vi "Data Queue Single.vi"(7 "Action":T1(ring), 8 "error in (no error)":errorcluster, 11 "Data In":sgl[][](array[numeric])) -> (0 "error out":errorcluster, 3 "Data Out":sgl[][](array[numeric]))   [LabVIEW 2017]
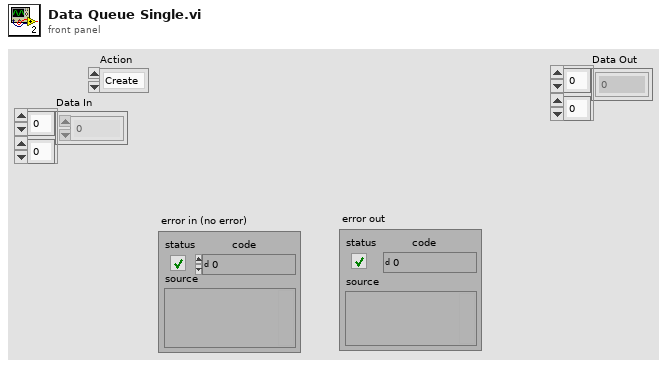
[diagram p1: front panel]
types:
  T1 = enum16{"Create", "Enqueue", "Dequeue", "Clear", "Release"}
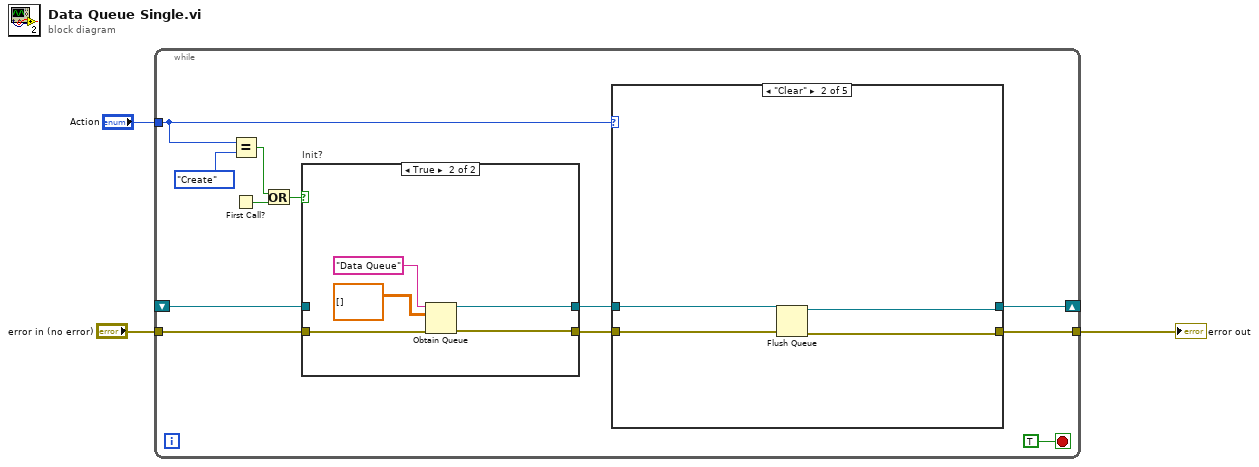
[diagram p0: block diagram]
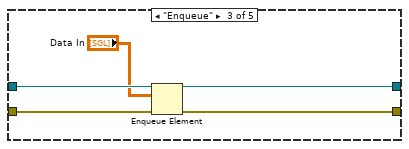
[diagram p4: hidden frame]
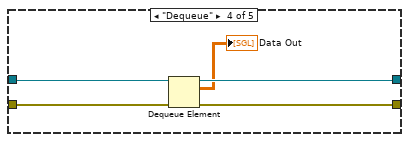
[diagram p5: hidden frame]
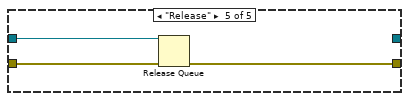
[diagram p6: hidden frame]
diagram:
  n1 = while {
    tunnel: "Action" -> [w14]
    tunnel: "error in (no error)" -> [w11]
    tunnel: [w9] -> w1
    shift-right: [w6] -> _
    shift-left: _ -> [w5]
    stop <- TRUE stop-if-true
    n2 = Equal?(x=w14, y=T1."Create") -> (x = y?=w13:bool)
    n3 = First Call?() -> (First Call?: T/F=w15:bool)
    n4 = Or(x=w13, y=w15) -> (x .or. y?=w12:bool)
    n5 = case "Init?" shown="True" w12 {
      tunnel: w11 -> [w17 w22]
      tunnel: [w17 w21] -> w10
      tunnel: [w16 w20] -> w7
      tunnel: w5 -> [w16 _]
      frame False {
      }
      frame True {
        n6 = Obtain Queue(name (unnamed)="Data Queue", element data type=sgl[][] [] ("Data In"), error in (no error)=w22) -> (queue out=w20:refnum<queue>, error out=w21:errorcluster)  [unwired: 2 in, 1 out]
      }
    }
    n7 = case shown="\"Clear\"" w14 {
      tunnel: w10 -> [w24 w28 w33 w38 w41]
      tunnel: [w24 w27 w32 w35 w40] -> w9
      tunnel: w7 -> [w23 w25 w30 w37 w39]
      tunnel: [w23 w26 w31 w36 _] -> w6
      frame "Create", Default {
      }
      frame "Clear" {
        n8 = Flush Queue(queue=w25, error in (no error)=w28) -> (queue out=w26:refnum<queue>, error out=w27:errorcluster)  [unwired: 1 out]
      }
      frame "Enqueue" {
        n9 = Enqueue Element(queue=w30, element="Data In", error in (no error)=w33) -> (queue out=w31:refnum<queue>, error out=w32:errorcluster)  [unwired: 2 out]
      }
      frame "Dequeue" {
        n10 = Dequeue Element(queue=w37, error in (no error)=w38) -> (queue out=w36:refnum<queue>, element=→"Data Out":sgl[][], error out=w35:errorcluster)  [unwired: 2 out]
      }
      frame "Release" {
        n11 = Release Queue(queue=w39, error in (no error)=w41) -> (error out=w40:errorcluster)  [unwired: 1 in, 2 out]
      }
    }
  }
  "error out" <- w1
